vi "WarningPopup.vi"(8 "error in (no error)":errorcluster, 11 "Error info":T1) -> (0 "error out":errorcluster, 3 "Select":enum16{"Ok", "Log", "Exit"}(ring))   [LabVIEW 2017, in "Error.lvlib"]
uses:
  Error.lvlib
  ctl/ErrorInfo.ctl
panel:
  in  "Log":bool
  in  "Kill":bool
  in  "OK":bool
  out "Error data":string
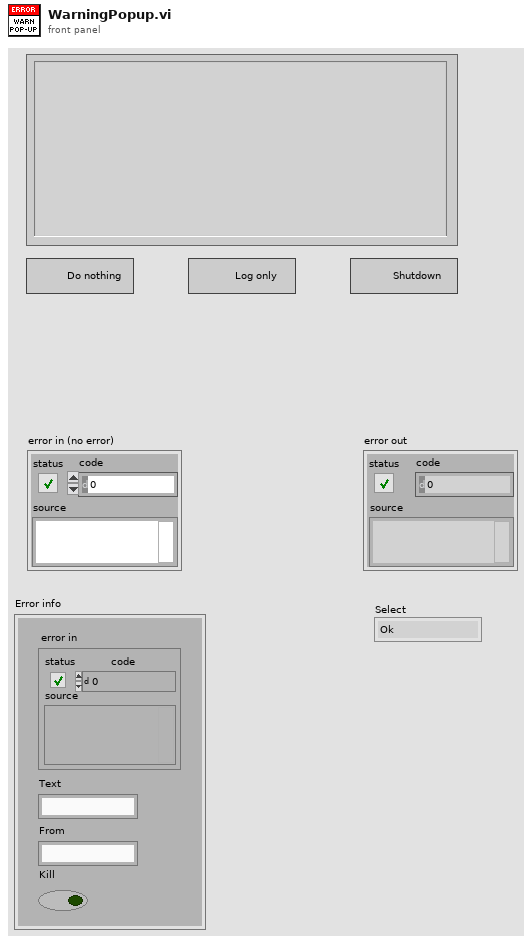
[diagram p1: front panel]
types:
  T1 = typedef "Error.lvlib/ErrorInfo.ctl" = cluster{"error in":errorcluster, "Text":string, "From":string, "Kill":bool}
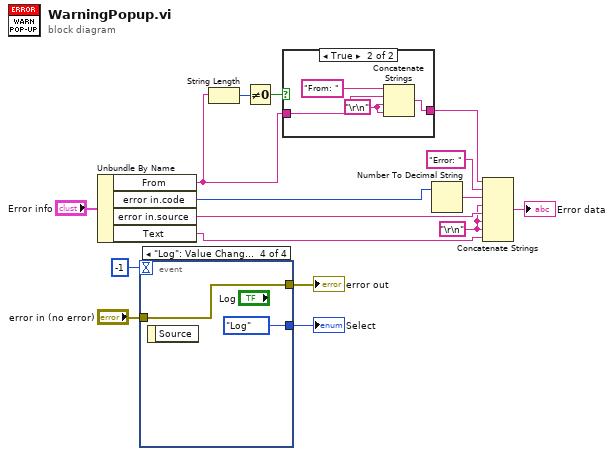
[diagram p0: block diagram]
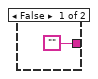
[diagram p2: hidden frame]
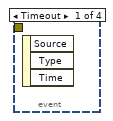
[diagram p3: hidden frame]
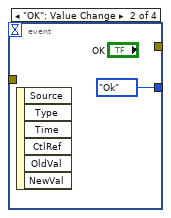
[diagram p4: hidden frame]
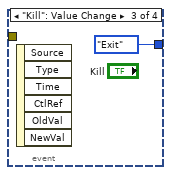
[diagram p5: hidden frame]
diagram:
  w3 = "\r\n"
  n1 = Unbundle By Name("Error info") -> ("From"=w9:string, "error in.code"=w6:i32, "error in.source"=w4:string, "Text"=w2:string)
  n2 = event shown="[3] \"Log\": Value Change" {
    selector: _ -> [_ _ _ _]
    dyn-events: _ -> [_ _ _ _]
    timeout: -1 -> [_ _ _ _]
    tunnel: "error in (no error)" -> [_ _ _ w19]
    tunnel: [_ enum16{"Ok", "Log", "Exit"}."Ok" ("Select") enum16{"Ok", "Log", "Exit"}."Exit" ("Select") enum16{"Ok", "Log", "Exit"}."Log" ("Select")] -> w14
    tunnel: [_ _ _ w19] -> w13
    event Timeout {
      n3 = event-data() -> ()  [unwired: 1 in, 3 out]
    }
    event "OK": Value Change {
      n4 = event-data() -> ()  [unwired: 1 in, 6 out]
    }
    event "Kill": Value Change {
      n5 = event-data() -> ()  [unwired: 1 in, 6 out]
    }
    event "Log": Value Change {
      n6 = event-data() -> ()  [unwired: 1 in, 1 out]
    }
  }
  "error out" <- w13
  "Select" <- w14
  n7 = String Length(string=w9) -> (length=w11:i32)
  n8 = Not Equal To 0?(x=w11) -> (x != 0?=w10:bool)
  n9 = case shown="True" w10 {
    tunnel: w9 -> [_ w25]
    tunnel: ["" w24] -> w8
    frame False {
    }
    frame True {
      w23 = "\r\n"
      n10 = Concatenate Strings("From: " ("string"), w25, w23, w23) -> (w24:string)
    }
  }
  n11 = Number To Decimal String(number=w6) -> (decimal integer string=w5:string)  [unwired: 1 in]
  n12 = Concatenate Strings(w8, "Error: " ("string"), w5, w3, w4, w3, w3, w2) -> (→"Error data":string)
